vi "m1m3_logEvent_CommandRejectionWarning.vi"(8 "error in (no error)":errorcluster, 11 "logevent_CommandRejectionWarning_Ctl":T1={"Timestamp"=0.0, "Command"="                                                                ", "Reason"="", "priority"=0}) -> (0 "error out":errorcluster, 2 "function return":i32, 3 "logevent_CommandRejectionWarning_Ctl out":T1={"Timestamp"=0.0, "Command"="                                                                ", "Reason"="", "priority"=0})   [LabVIEW 2016, in "SALLV_m1m3.lvlib"]
doc: "int m1m3_shm_logEvent_CommandRejectionWarningLV(m1m3_logevent_CommandRejectionWarningLV *logevent_CommandRejectionWarning_Ctl );"
uses:
  SALLV_m1m3.lvlib
  DataTypes/logevent_CommandRejectionWarning.ctl
  SALLV_m1m3.so
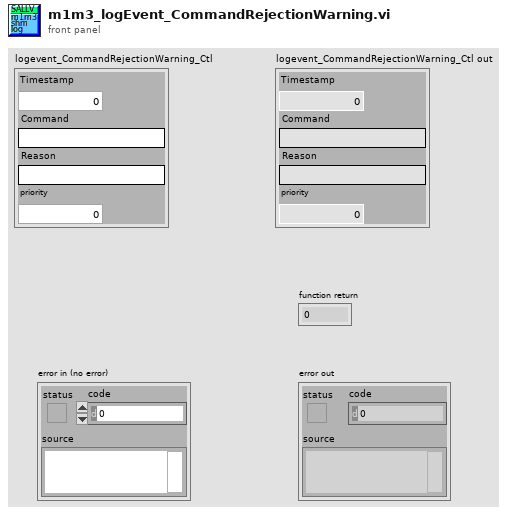
[diagram p1: front panel]
types:
  T1 = typedef "SALLV_m1m3.lvlib/logevent_CommandRejectionWarning.ctl" = cluster{"Timestamp":dbl, "Command":string, "Reason":string, "priority":i32}
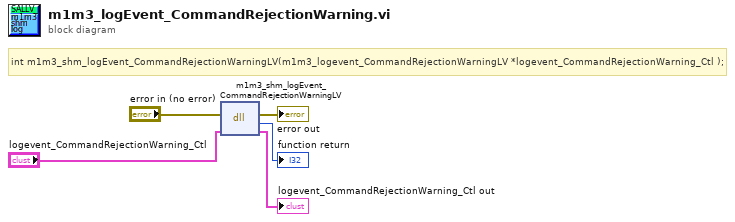
[diagram p0: block diagram]
diagram:
  # "int m1m3_shm_logEvent_CommandRejectionWarningLV(m1m3_logevent_CommandRejectionWarningLV *logevent_CommandRejectionWarning_Ctl );"
  n1 = dll-call lib="opt/CODE/SALLV_m1m3/SALLV_m1m3.*" fn="m1m3_shm_logEvent_CommandRejectionWarningLV"(error in="error in (no error)", "logevent_CommandRejectionWarning_Ctl"="logevent_CommandRejectionWarning_Ctl") -> (error out=→"error out":errorcluster, →"function return":i32, "logevent_CommandRejectionWarning_Ctl"=→"logevent_CommandRejectionWarning_Ctl out":T1)  [unwired: 2 in, 1 out]
